vi "Screen_Vitreous.vi"(5 "File to Process":path) -> ()   [LabVIEW 2022 SP3]
uses:
  ViewData/-ReadEye/ScaleMethod.ctl
  <vilib>/Utility/miscctls.llb/LVOffsetAndMultiplierTypeDef.ctl
  <vilib>/Utility/miscctls.llb/LVRectTypeDef.ctl
  <vilib>/Utility/miscctls.llb/LVBoundsTypeDef.ctl
  <vilib>/Analysis/5stat.llb/RMS (DBL).vi
  <vilib>/Analysis/NI_AALPro.lvlib
panel:
  out "Current File#":i32
  out "Total #Files":i32
  in  "Next File in Dir?":bool caption="F1"
  in  "Prev File":bool caption="F2"
  in  "Delete File":bool caption="<Delete>"
  in  "Tab Control":enum32{"Images", "Misc"}(tab)
  out "dB":dbl[][](graph)
  out "Sector":dbl[][](graph)
  in  "Slide":cluster{dbl, dbl}(slide)={0.0, -48.10126582278481} scale=-80.0..-1.0
  in  "Comment Field (Optional)":string
  in  "Save Comment ?":bool
  in  "Type of Mean":u16(ring)=4 items=["Mean from lines", "Mean just lines", "Poly Mean", "No mean", "Filter"]
  in  "Filter Prams":T1={"low cutoff"=5, "order"=81, "high cutoff"=35}
  in  "Sound Speed":i16=1485
  out "RMS noise":dbl format="%#.2g"
  out "DynRange":dbl format="%#.2f"
  out "RF Window Pts":i32
  out "RF Lines":i32
  in  "Axis scaling":bool=TRUE
  in  "View Header?":bool
  in  "Alter Header":bool
  in  "Eye to BMP":bool
  in  "Display mode":T2=enum."dB Scale"
  out "Raw data":dbl[][](graph)
  out "Scan Info":T3
  in  "Create Sector":bool
  out "Axis scaling Params":T4 {"Y high" format="%.2f"; "Y low" format="%.2f"; "X left" format="%.2f"; "X right" format="%.2f"}
  out "cursor":dbl
  in  "Smooth factor":i32=1
  in  "Pixels in x":i16=170
  in  "Pixels in y":i16=1000
  in  "Reduce x data factor":i32=2
  out "inc x (mm)":dbl format="%.3f"
  out "inc y (mm)":dbl format="%.3f"
  in  "Add Lines":u16=1
  in  "File Ext":string="*.eye"
  in  "Save eye":bool
  in  "ExitSendCmd":bool
  # "For screening *.eye file stacks. Mainly meant for Aviso data acquired with custom digitizer set up."
  # "Push folder symbol to select first 'eye' to view in a folder.\nPress \"F1\" on keybard to increment up one image\nPress \"F2\" on keyboard to decrement down one image\nPress \"<Delete>\" on keyboard to delete a \"bad\" image\nSelect \"Save Comment\" to save any text that is entered into \"Comment Field\"\nExit program by pressing \"Stop\""
  # "© 2022 Weill Cornell Medicine"
  # "Crop sides with yellow line"
  # "Save sector as *.eye file in virtual RF space. Use add lines 4.\nPixels in y adjusts virtual sampling rate."
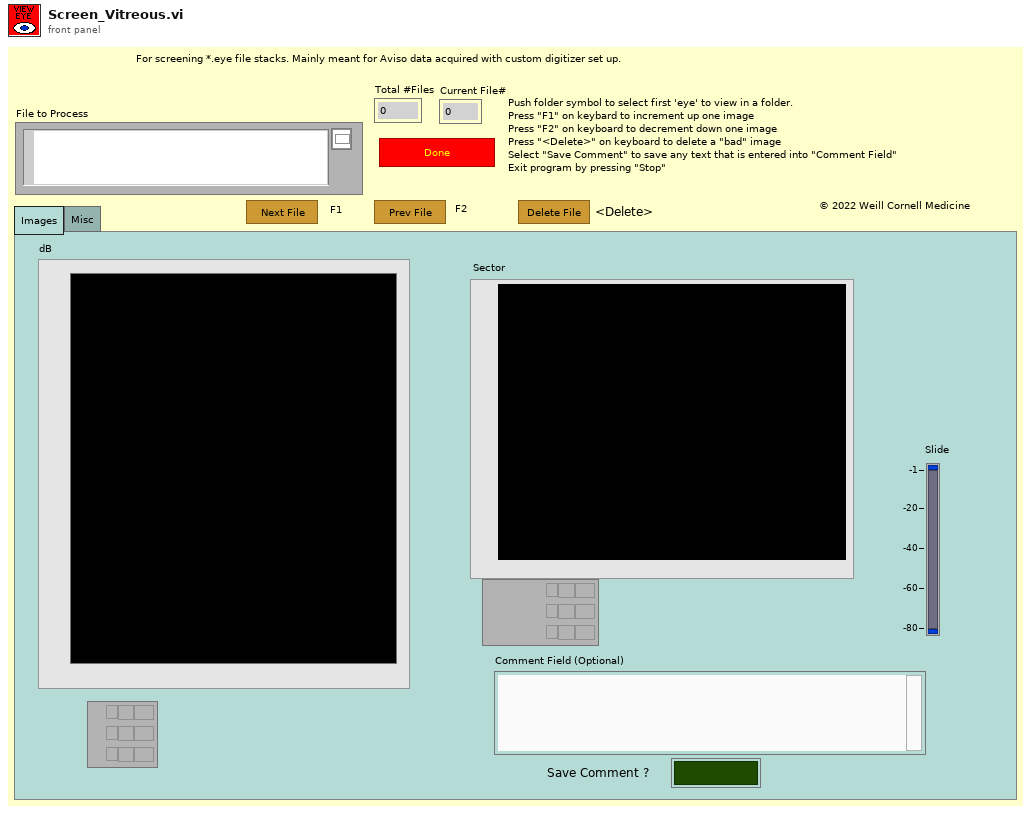
[diagram p1: front panel]
types:
  T1 = cluster{"low cutoff":i32, "order":i32, "high cutoff":i32}
  T2 = typedef "ScaleMethod.ctl" = enum16{"Linear Abs Grey", "Log Grey Scale", "Linear Color Scale", "dB Scale", "Verasonics Doppler"}
  T3 = cluster{"delay":sgl, "pivot distance":sgl, "sector scan angle":sgl, "operator":string, "Scan Mode":string, "location":string}
  T4 = cluster{"X right":dbl, "X left":dbl, "Y low":dbl, "Y high":dbl}
  T5 = enum16{"big-endian, network order", "native, host order", "little-endian"}
  T6 = enum16{"open", "replace", "create", "open or create", "replace or create", "replace or create with confirmation"}
  T7 = typedef "Header.ctl" = cluster{"header info":cluster{"Header":string, "Head length":i16}, "A/D info":cluster{"# rf points per line":u16, "# lines per scan":u16, "sample rate MHz":u16, "# A/D bits":i16, "# bytes per A/D":u16, "TGC Flag":u16, "A/D Type":string}, "Tranducer Info":cluster{"bandwidth":sgl, "center freq":sgl, "start freq":sgl, "ID":i32}, "Scan Info":cluster{"delay":sgl, "pivot distance":sgl, "sector scan angle":sgl, "operator":string, "Scan Mode":string, "location":string}, "Time/Date Info":cluster{"date":string, "time":string}, "RF Info":cluster{"RF file name":string, "RF file att":string, "RF cal file name":string, "RF cal file att":string}, "Patient Info":cluster{"ID":string, "extended ID":string, "age":u16, "sex":string, "previously\nscanned":string, "PSA":sgl, "LOS":u8, "Ethnicty 2":u8, "Race":u8}, "Tissue Type":cluster{"organ":i16, "disease type":i16, "disease location":i16, "IQ_pts":u16, "RcvBuffer":u8, "RcvFrame":u16, "IQBuff":u8, "IQFrame":u16, "IQPage":u8}, "Votage scaling":cluster{"Digitizer (dB)":sgl, "Gain (dB)":sgl, "Atten (dB)":sgl}, "Comment":string, "Misc Info":cluster{"avg num":u16, "c speed":i16, "Div By or SF zones":i16, "XMIT CHS":u8, "RCV CHS":u8, "Xmit angle":sgl}, "Therapy Parameters":cluster{"Theraputic Freq (MHz)":sgl, "Time on (s)":sgl, "Therapy amplitude (mV)":sgl, "Lines Before":u16, "Lines After":u16}, "Scan Settings":cluster{"Energy (uJ or V)":u8, "Damp (Ohm) or Fc":u8, "HP Filt (KHz)":u8, "LP Filt (MHz)":u8, "Gain (db)":u8, "prf (kHz)":sgl, "Distance between\nscan lines (um)":u16, "Distance between\nscan planes (um)":u16, "Scan line gap (um)":sgl, "Scan plane gap (um)":sgl}, "Compression Parameters":cluster{"F1 (MHz)":sgl, "F2 (MHz)":sgl, "% taper":sgl, "duration":sgl}, "Patient Info Xtra":cluster{"First Name":string, "Last Name":string, "Notes":string}, "ROI Box":u16[]}
  T8 = typedef "LVOffsetAndMultiplierTypeDef.ctl" = cluster{"Offset":dbl, "Multiplier":dbl}
  T9 = typedef "LVBoundsTypeDef.ctl" = cluster{"Width":u32, "Height":u32}
  T10 = typedef "LVRectTypeDef.ctl" = cluster{"Left":i16, "Top":i16, "Right":i16, "Bottom":i16}
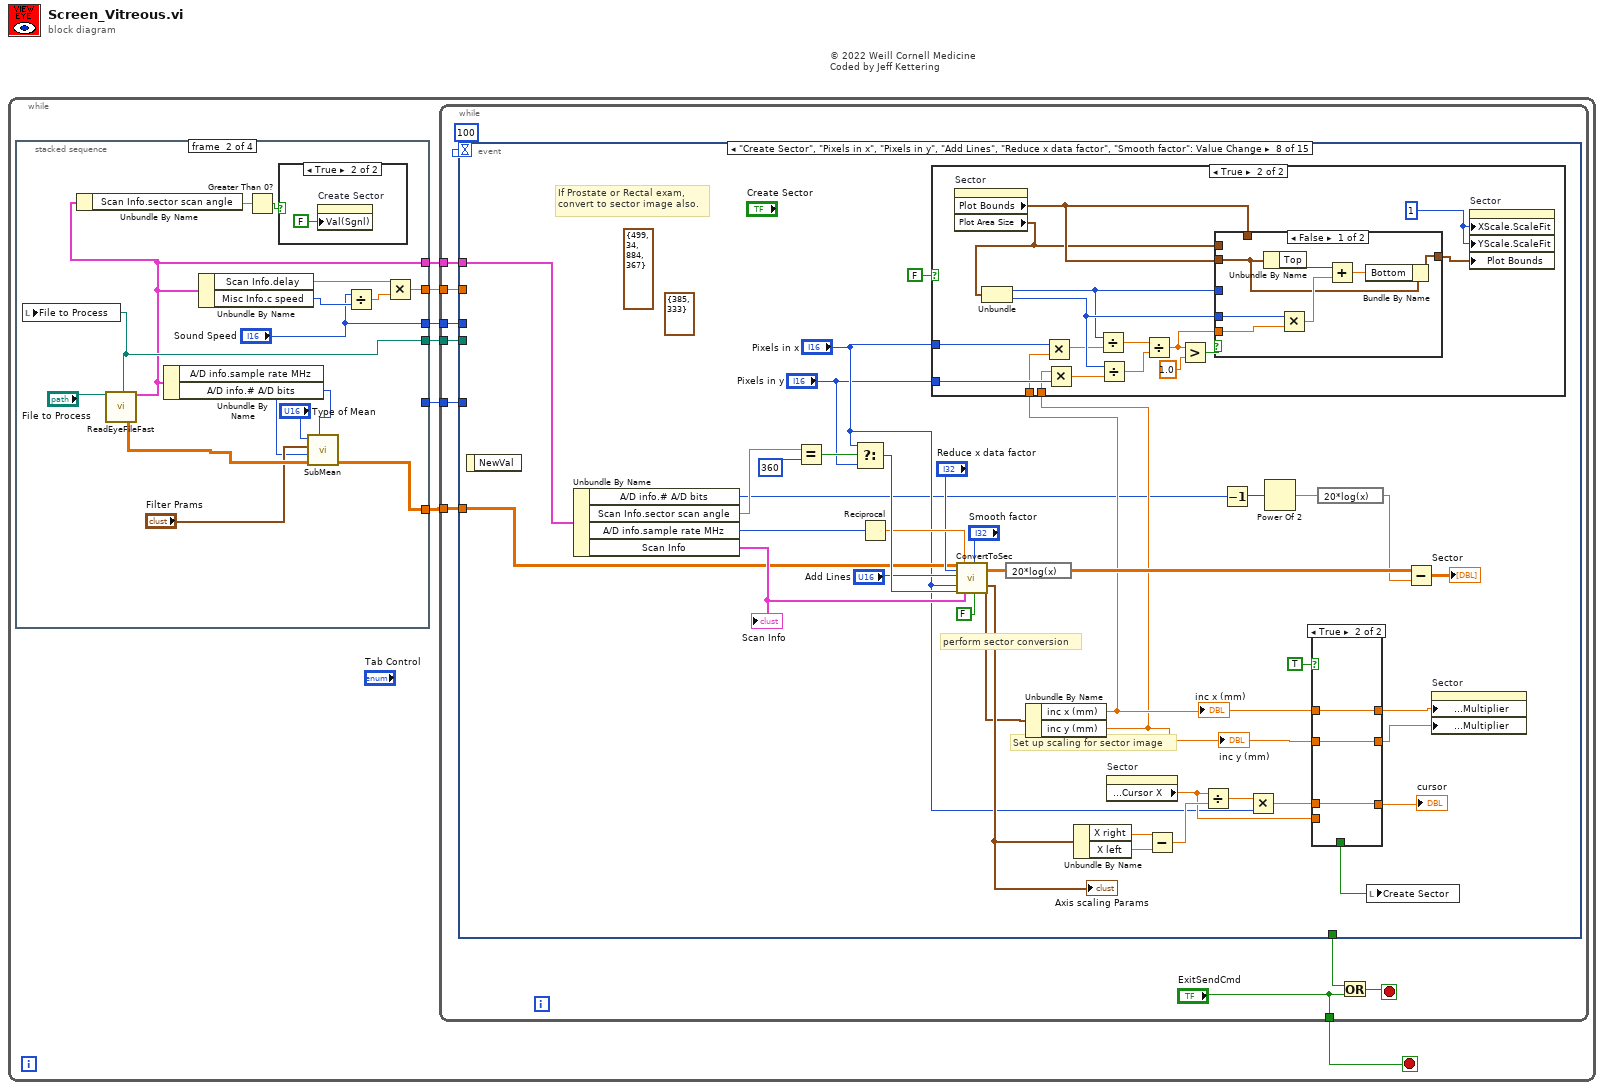
[diagram p0: block diagram]
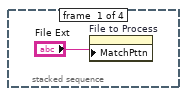
[diagram p2: hidden frame]
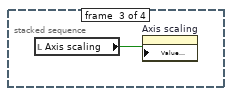
[diagram p4: hidden frame]
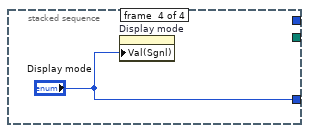
[diagram p5: hidden frame]
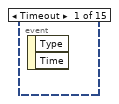
[diagram p6: hidden frame]
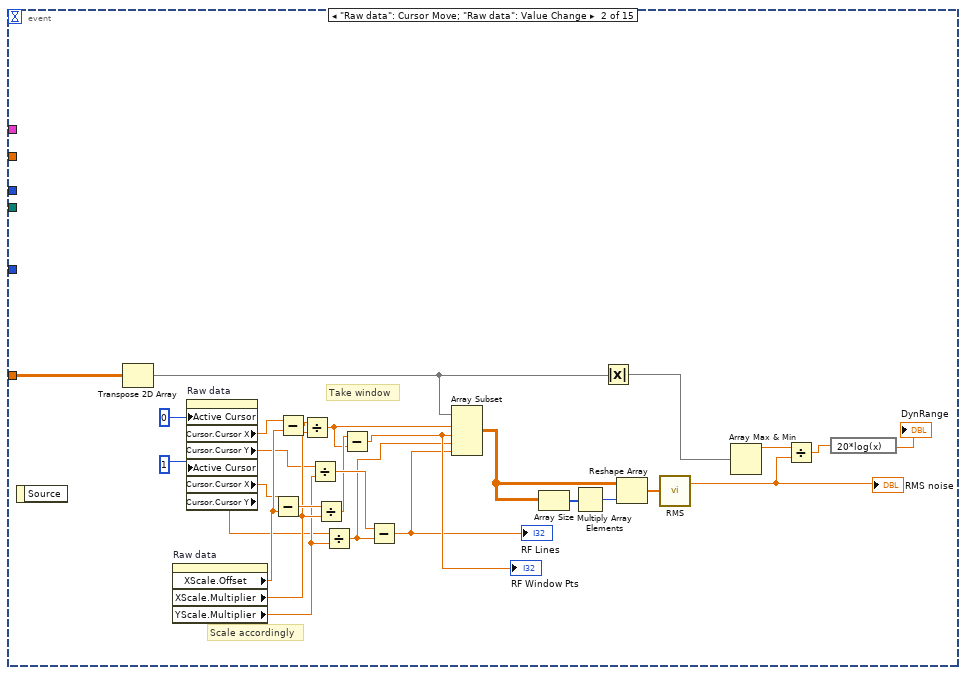
[diagram p7: hidden frame]
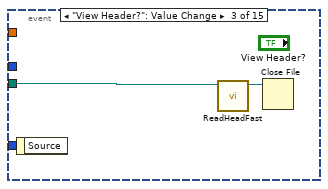
[diagram p8: hidden frame]
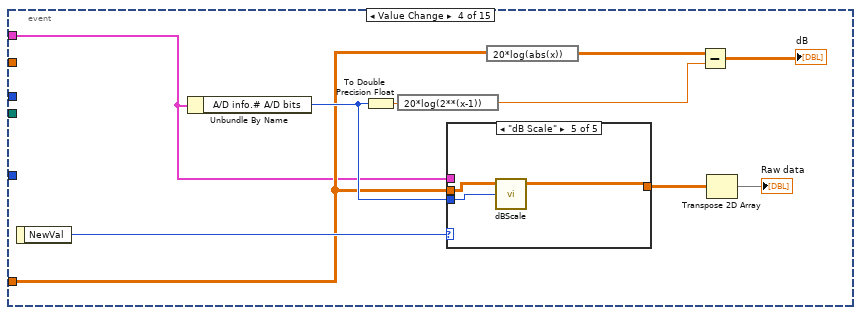
[diagram p9: hidden frame]
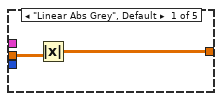
[diagram p10: hidden frame]
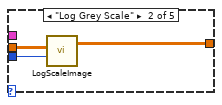
[diagram p11: hidden frame]
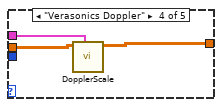
[diagram p13: hidden frame]
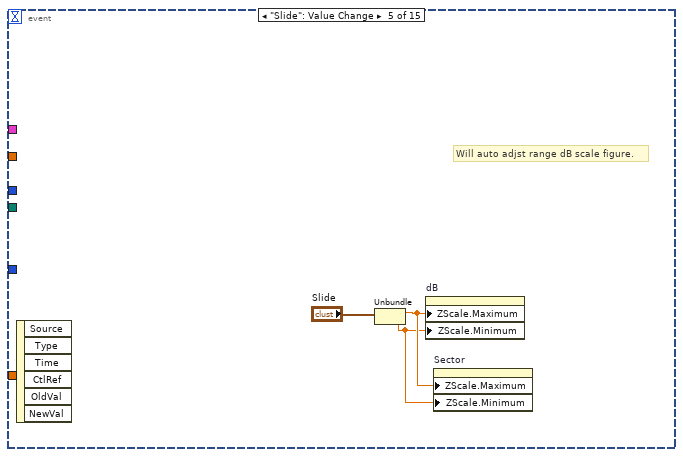
[diagram p14: hidden frame]
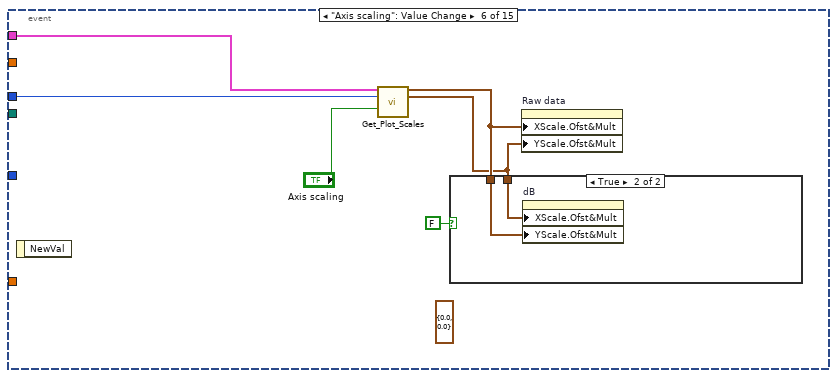
[diagram p15: hidden frame]
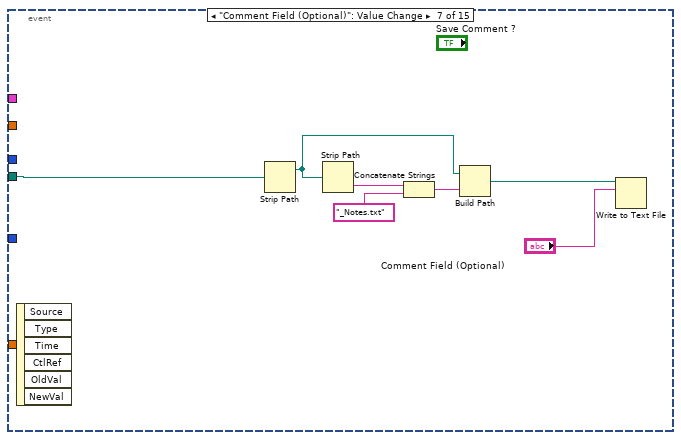
[diagram p17: hidden frame]
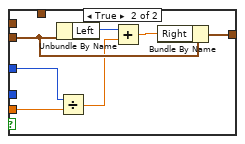
[diagram p19: hidden frame]
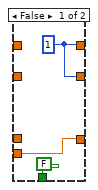
[diagram p20: hidden frame]
diagram:
  # "© 2022 Weill Cornell Medicine\nCoded by Jeff Kettering"
  n1 = while {
    stop <- w6 stop-if-true
    n2 = stacked-sequence {
      tunnel: [_ w22 _ _] -> w7
      tunnel: [_ w24 _ _] -> w5
      tunnel: [_ _ _ "Display mode"] -> w4
      tunnel: [_ w10 _ _] -> w3
      tunnel: [_ w15 _ _] -> w2
      tunnel: [_ "Sound Speed" _ _] -> w1
      frame #0 {
        n3 = property on="File to Process" class="Path"("MatchPttn"="File Ext") -> ()  [unwired: 2 in, 2 out]
      }
      frame #1 {
        n4 = call "ReadEyeFileFast.vi"("new file path"="File to Process") -> ("new path out"=w24:path, "2-D data array"=w23:sgl[][], "Header In"=w10:T7)  [unwired: 1 in, 15 out]
        n5 = local write "File to Process"(w24) -> ()
        n6 = Unbundle By Name(w10) -> ("Scan Info.sector scan angle"=w11:sgl)
        n7 = Unbundle By Name(w10) -> ("A/D info.sample rate MHz"=w13:u16, "A/D info.# A/D bits"=w9:i16)
        n8 = Unbundle By Name(w10) -> ("Scan Info.delay"=w16:sgl, "Misc Info.c speed"=w18:i16)
        n9 = Greater Than 0?(x=w11) -> (x > 0?=w12:bool)
        n10 = case shown="True" w12 {
          frame False {
          }
          frame True {
            n11 = property on="Create Sector" class="Bool (strict)"("Val(Sgnl)"=FALSE ("Value (Signaling)")) -> ()  [unwired: 2 in, 2 out]
          }
        }
        n12 = call "SubMean.vi"("Bit Depth"=w9, "Scan Data In"=w23, "Samp Rate (MHz)"=w13, "Filter Prams"="Filter Prams", "Type of Mean"="Type of Mean") -> ("Array"=w22:dbl[][])  [unwired: 1 in, 2 out]
        n13 = Divide(x="Sound Speed", y=w18) -> (x/y=w17:dbl)
        n14 = Multiply(x=w16, y=w17) -> (x*y=w15:dbl)
      }
      frame #2 {
        n15 = local read "Axis scaling"() -> (w26:bool)
        n16 = property on="Axis scaling" class="Bool (strict)"("Value (Signaling)"=w26) -> ()  [unwired: 2 in, 2 out]
      }
      frame #3 {
        n17 = property on="Display mode" class="Enum (strict)"("Val(Sgnl)"="Display mode") -> ()  [unwired: 2 in, 2 out]
      }
    }
    n18 = while {
      tunnel: w7 -> [w37]
      tunnel: w5 -> [w35]
      tunnel: w4 -> [w34]
      tunnel: ["ExitSendCmd"] -> w6
      tunnel: w3 -> [w30]
      tunnel: w2 -> [w29]
      tunnel: w1 -> [w28]
      stop <- w31 stop-if-true
      n19 = event shown="[7] \"Create Sector\", \"Pixels in x\", \"Pixels in y\", \"Add Lines\", \"Reduce x data factor\", \"Smooth factor\": Value Change" {
        selector: _ -> [_ _ _ _ _ _ _ _ _ _ _ _ _ _ _]
        dyn-events: _ -> [_ _ _ _ _ _ _ _ _ _ _ _ _ _ _]
        timeout: 100 -> [_ _ _ _ _ _ _ _ _ _ _ _ _ _ _]
        tunnel: w37 -> [_ w57 _ w72 _ _ _ w118 w226 _ _ _ _ _ _]
        tunnel: w35 -> [_ _ w67 _ _ _ w107 _ w205 _ w246 w294 w307 w309 _]
        tunnel: w34 -> [_ _ _ _ _ _ _ _ _ _ _ _ _ _ _]
        tunnel: [_ _ _ _ _ _ _ _ _ TRUE TRUE TRUE TRUE _ TRUE] -> w32
        tunnel: w30 -> [_ _ _ w70 _ w96 _ w131 w215 _ _ _ _ _ _]
        tunnel: w29 -> [_ _ _ _ _ _ _ _ _ _ _ _ _ _ _]
        tunnel: w28 -> [_ _ _ _ _ w97 _ _ _ _ _ _ _ _ _]
        event Timeout {
          n20 = event-data() -> ()  [unwired: 3 out]
        }
        event "Raw data": Cursor Move; "Raw data": Value Change {
          # "Take window"
          # "Scale accordingly"
          n21 = event-data() -> ()  [unwired: 2 out]
          n22 = Transpose 2D Array(2D array=w57) -> (transposed array=w42:dbl[][])
          n23 = property on="Raw data" class="IntGraph (strict)"() -> ("XScale.Offset"=w56:dbl, "XScale.Multiplier"=w55:dbl, "YScale.Multiplier"=w54:dbl)  [unwired: 2 in, 2 out]
          n24 = property on="Raw data" class="IntGraph (strict)"("Active Cursor"=u32 0 ("Write Attribute"), "Active Cursor"=u32 1 ("Write Attribute")) -> ("Cursor.Cursor X"=w53:dbl, "Cursor.Cursor Y"=w49:dbl, "Cursor.Cursor X"=w52:dbl, "Cursor.Cursor Y"=w48:dbl)  [unwired: 2 in, 2 out]
          n25 = Subtract(x=w52, y=w56) -> (x-y=w59:dbl)
          n26 = Subtract(x=w53, y=w56) -> (x-y=w60:dbl)
          n27 = Divide(x=w60, y=w55) -> (x/y=w47:dbl)
          n28 = Divide(x=w49, y=w54) -> (x/y=w61:dbl)
          n29 = Divide(x=w59, y=w55) -> (x/y=w58:dbl)
          n30 = Divide(x=w48, y=w54) -> (x/y=w45:dbl)
          n31 = Subtract(x=w58, y=w47) -> (x-y=w46:dbl)
          "RF Window Pts" <- w46
          n32 = Subtract(x=w61, y=w45) -> (x-y=w44:dbl)
          "RF Lines" <- w44
          n33 = Array Subset(array=w42, index (row)=w47, length (row)=w46, index (col)=w45, length (col)=w44) -> (w39:dbl[][])
          n34 = Array Size(array=w39) -> (size(s)=w64:i32[])
          n35 = Multiply Array Elements(1:w64) -> (0:w62:i32)
          n36 = Absolute Value(x=w42) -> (abs(x)=w43:dbl[][])
          n37 = Reshape Array(w39, w62) -> (w63:dbl[])
          n38 = call-poly <vilib>:"RMS.vi"("X"=w63) -> ("rms value"=w38:dbl)  [unwired: 1 out]
          "RMS noise" <- w38
          n39 = Array Max & Min(array=w43) -> (max value=w65:dbl)  [unwired: 3 out]
          n40 = Divide(x=w65, y=w38) -> (x/y=w40:dbl)
          n41 = expression code="20*log(x)"(w40) -> (→"DynRange":dbl)
        }
        event "View Header?": Value Change {
          n42 = event-data() -> ()  [unwired: 2 out]
          n43 = call "ReadHeadFast.vi"("new file path"=w67) -> ("refnum out"=w66:refnum<file>)  [unwired: 7 in, 3 out]
          n44 = Close File(refnum=w66) -> ()  [unwired: 1 in, 2 out]
        }
        event Value Change {
          n45 = event-data() -> ("NewVal"=w76:T2)  [unwired: 1 out]
          n46 = Unbundle By Name(w70) -> ("A/D info.# A/D bits"=w75:i16)
          n47 = To Double Precision Float(number=w75) -> (double precision float=w74:dbl)
          n48 = expression code="20*log(2**(x-1))"(w74) -> (w73:dbl)
          n49 = case shown="\"dB Scale\"" w76 {
            tunnel: [w78 w82 w83 w85 w88] -> w69
            tunnel: w72 -> [w79 w81 w83 w86 w89]
            tunnel: w75 -> [_ w80 _ _ w87]
            tunnel: w70 -> [_ _ _ w84 _]
            frame "Linear Abs Grey", Default {
              n50 = Absolute Value(x=w79) -> (abs(x)=w78:dbl[][])
            }
            frame "Log Grey Scale" {
              n51 = call "LogScaleImage.vi"("A/D bits"=w80, "input array"=w81) -> ("log scale image"=w82:dbl[][])  [unwired: 1 out]
            }
            frame "Linear Color Scale" {
            }
            frame "Verasonics Doppler" {
              n52 = call "DopplerScale.vi"("Header In"=w84, "Velocity index in"=w86) -> ("Velocity Out"=w85:dbl[][])  [unwired: 6 in, 3 out]
            }
            frame "dB Scale" {
              n53 = call "dBScale.vi"("Bit Depth"=w87, "Data In"=w89) -> ("Data Out"=w88:dbl[][])  [unwired: 3 in]
            }
          }
          n54 = expression code="20*log(abs(x))"(w72) -> (w71:dbl[][])
          n55 = Subtract(x=w71, y=w73) -> (x-y=→"dB":dbl[][])
          n56 = Transpose 2D Array(2D array=w69) -> (transposed array=→"Raw data":dbl[][])
        }
        event "Slide": Value Change {
          # "Will auto adjst range dB scale figure."
          n57 = event-data() -> ()  [unwired: 7 out]
          n58 = Unbundle("Slide") -> (w91:dbl, w90:dbl)
          n59 = property on="dB" class="IntGraph (strict)"("ZScale.Maximum"=w91, "ZScale.Minimum"=w90) -> ()  [unwired: 2 in, 2 out]
          n60 = property on="Sector" class="IntGraph (strict)"("ZScale.Maximum"=w91, "ZScale.Minimum"=w90) -> ()  [unwired: 2 in, 2 out]
        }
        event "Axis scaling": Value Change {
          (unwired) T8 {"Offset"=0.0, "Multiplier"=0.0} ("X Scale.Offset and Multiplier")
          n61 = event-data() -> ()  [unwired: 2 out]
          n62 = call "Get_Plot_Scales.vi"("Header In"=w96, "Sound Speed modify"=w97, "Axis scaling"="Axis scaling") -> ("Depth Scale"=w95:cluster{"start depth":dbl, "depth interval":dbl}, "Width Scale"=w94:cluster{"Start":dbl, "width Interval":dbl})  [unwired: 11 in]
          n63 = case shown="True" FALSE {
            tunnel: w95 -> [_ w100]
            tunnel: w94 -> [_ w99]
            frame False {
            }
            frame True {
              n64 = property on="dB" class="IntGraph (strict)"("XScale.Ofst&Mult"=w99, "YScale.Ofst&Mult"=w100) -> ()  [unwired: 2 in, 2 out]
            }
          }
          n65 = property on="Raw data" class="IntGraph (strict)"("XScale.Ofst&Mult"=w95, "YScale.Ofst&Mult"=w94) -> ()  [unwired: 2 in, 2 out]
        }
        event "Comment Field (Optional)": Value Change {
          n66 = event-data() -> ()  [unwired: 7 out]
          n67 = Strip Path(path=w107) -> (stripped path=w101:path)  [unwired: 1 out]
          n68 = Strip Path(path=w101) -> (name=w106:string)  [unwired: 1 out]
          n69 = Concatenate Strings(w106, "_Notes.txt" ("search string")) -> (w102:string)
          n70 = Build Path(base path=w101, name or relative path=w102) -> (appended path=w104:path)
          n71 = Write to Text File(file (use dialog)=w104, text="Comment Field (Optional)") -> ()  [unwired: 2 in, 3 out]
        }
        event "Create Sector", "Pixels in x", "Pixels in y", "Add Lines", "Reduce x data factor", "Smooth factor": Value Change {
          (unwired) T9 {"Width"=385, "Height"=333} ("Plot Area:Size")
          (unwired) T10 {"Left"=499, "Top"=34, "Right"=884, "Bottom"=367} ("Plot Area Bounds")
          # "Set up scaling for sector image"
          # "If Prostate or Rectal exam,\nconvert to sector image also."
          # "perform sector conversion"
          n72 = event-data() -> ()  [unwired: 2 out]
          n73 = Unbundle By Name(w131) -> ("A/D info.# A/D bits"=w110:i16, "Scan Info.sector scan angle"=w123:sgl, "A/D info.sample rate MHz"=w124:u16, "Scan Info"=w130:T3)
          "Scan Info" <- w130
          n74 = Equal?(x=w123, y=360) -> (x = y?=w143:bool)
          n75 = Select(t="Pixels in x", s=w143, f="Pixels in y") -> (s? t:f=w145:i16)
          n76 = Reciprocal(x=w124) -> (1/x=w142:dbl)
          n77 = call "ConvertToSec.vi"("raw image data in"=w118, "reduce pts by factor of"="Reduce x data factor", "Add Lines"="Add Lines", "pixels in x"="Pixels in x", "pixels in y"=w145, "Time between rf pts\nmicros"=w142, "Scan Info"=w130, "Smooth factor"="Smooth factor", "use min z value?"=FALSE) -> ("raw sector out"=w121:dbl[][], "Axis scaling Params"=w132:T4, "scales"=w128:cluster{"inc x (mm)":dbl, "inc y (mm)":dbl})  [unwired: 3 in, 5 out]
          "Axis scaling Params" <- w132
          n78 = expression code="20*log(x)"(w121) -> (w120:dbl[][])
          n79 = Unbundle By Name(w128) -> ("inc x (mm)"=w115:dbl, "inc y (mm)"=w114:dbl)
          "inc y (mm)" <- w114
          "inc x (mm)" <- w115
          n80 = case shown="True" FALSE {
            tunnel: "Pixels in x" -> [_ w153]
            tunnel: "Pixels in y" -> [_ w152]
            tunnel: w115 -> [_ w151]
            tunnel: w114 -> [_ w150]
            frame False {
            }
            frame True {
              w148 = u8 1 ("X Scale.Scale Fit")
              n81 = property on="Sector" class="IntGraph (strict)"() -> ("Plot Bounds"=w147:T10, "Plot Area Size"=w146:T9)  [unwired: 2 in, 2 out]
              n82 = Unbundle(w146) -> ("Width"=w160:u32, "Height"=w162:u32)
              n83 = Multiply(x=w153, y=w151) -> (x*y=w154:dbl)
              n84 = Multiply(x=w150, y=w152) -> (x*y=w155:dbl)
              n85 = Divide(x=w160, y=w154) -> (x/y=w156:dbl)
              n86 = Divide(x=w162, y=w155) -> (x/y=w157:dbl)
              n87 = Divide(x=w156, y=w157) -> (x/y=w161:dbl)
              n88 = Greater?(x=w161, y=1.0) -> (0:w158:bool)
              n89 = case shown="False" w158 {
                tunnel: w160 -> [_ w176]
                tunnel: w161 -> [w169 w175]
                tunnel: w162 -> [w168 _]
                tunnel: w147 -> [w163 w174]
                tunnel: [w164 w170] -> w149
                tunnel: w147 -> [_ _]
                tunnel: w146 -> [_ _]
                frame False {
                  n90 = Unbundle By Name(w163) -> ("Top"=w167:i16)
                  n91 = Multiply(x=w168, y=w169) -> (x*y=w165:dbl)
                  n92 = Add(x=w167, y=w165) -> (x+y=w166:dbl)
                  n93 = Bundle By Name(cluster=w163, "Bottom"=w166) -> (w164:T10)
                }
                frame True {
                  n94 = Unbundle By Name(w174) -> ("Left"=w172:i16)
                  n95 = Divide(x=w176, y=w175) -> (x/y=w173:dbl)
                  n96 = Add(x=w172, y=w173) -> (x+y=w171:dbl)
                  n97 = Bundle By Name(cluster=w174, "Right"=w171) -> (w170:T10)
                }
              }
              n98 = property on="Sector" class="IntGraph (strict)"("XScale.ScaleFit"=w148, "YScale.ScaleFit"=w148, "Plot Bounds"=w149) -> ()  [unwired: 2 in, 2 out]
            }
          }
          n99 = Unbundle By Name(w132) -> ("X right"=w141:dbl, "X left"=w140:dbl)
          n100 = property on="Sector" class="IntGraph (strict)"() -> ("Cursor.Cursor Position:Cursor X"=w134:dbl)  [unwired: 2 in, 2 out]
          n101 = Subtract(x=w141, y=w140) -> (x-y=w139:dbl)
          n102 = Divide(x=w134, y=w139) -> (x/y=w138:dbl)
          n103 = Decrement(x=w110) -> (x-1=w112:i16)
          n104 = Multiply(x=w138, y="Pixels in x") -> (x*y=w135:dbl)
          n105 = Power Of 2(x=w112) -> (2^x=w111:dbl)
          n106 = case shown="True" TRUE {
            tunnel: w115 -> [_ w182]
            tunnel: [w179 w182] -> w137
            tunnel: [w179 w181] -> w136
            tunnel: w114 -> [_ w181]
            tunnel: w135 -> [_ w180]
            tunnel: [w178 w180] -> w133
            tunnel: w134 -> [w178 _]
            tunnel: [FALSE ("Create Sector") _] -> w119
            frame False {
              w179 = 1
            }
            frame True {
            }
          }
          "cursor" <- w133
          n107 = expression code="20*log(x)"(w111) -> (w109:dbl)
          n108 = local write "Create Sector"(w119) -> ()
          n109 = Subtract(x=w120, y=w109) -> (x-y=→"Sector":dbl[][])
          n110 = property on="Sector" class="IntGraph (strict)"("X Scale.Offset and Multiplier:Multiplier"=w137, "Y Scale.Offset and Multiplier:Multiplier"=w136) -> ()  [unwired: 2 in, 2 out]
        }
        event "Save eye": Value Change {
          w207 = FALSE ("prepend array or string size? (T)")
          w214 = sgl 0.0 ("Scan Info.pivot distance")
          # "Set up scaling for sector image"
          # "perform sector conversion"
          n111 = event-data() -> ()  [unwired: 7 out]
          n112 = Unbundle By Name(w215) -> ("Scan Info.sector scan angle"=w227:sgl, "A/D info.sample rate MHz"=w228:u16, "Scan Info"=w231:T3, "Misc Info.c speed"=w197:i16)
          n113 = local read "Pixels in y"() -> (w225:i16)
          n114 = local read "Pixels in x"() -> (w211:i16)
          n115 = Equal?(x=w227, y=360) -> (x = y?=w234:bool)
          n116 = Select(t=w211, s=w234, f=w225) -> (s? t:f=w210:i16)
          n117 = Reciprocal(x=w228) -> (1/x=w233:dbl)
          n118 = Strip Path(path=w205) -> (stripped path=w190:path, name=w204:string)
          n119 = local read "Add Lines"() -> (w223:u16)
          n120 = local read "Reduce x data factor"() -> (w224:i32)
          n121 = local read "Smooth factor"() -> (w191:i32)
          n122 = call "ConvertToSec.vi"("raw image data in"=w226, "reduce pts by factor of"=w224, "Add Lines"=w223, "pixels in x"=w211, "pixels in y"=w210, "Time between rf pts\nmicros"=w233, "Scan Info"=w231, "Abs?"=FALSE, "Interp Mode"=2, "Smooth factor"=w191, "use min z value?"=FALSE) -> ("raw sector out"=w206:dbl[][], "Axis scaling Params"=w232:T4, "scales"=w229:cluster{"inc x (mm)":dbl, "inc y (mm)":dbl})  [unwired: 1 in, 5 out]
          n123 = Search and Replace String(input string=w204, search string=".eye" ("input string"), replace string="Sec.eye" ("replace string (\"\")")) -> (result string=w203:string)  [unwired: 5 in, 3 out]
          n124 = Build Path(base path=w190, name or relative path="Sector" ("replace string (\"\")")) -> (appended path=w187:path)
          n125 = Unbundle By Name(w229) -> ("inc x (mm)"=w199:dbl, "inc y (mm)"=w196:dbl)
          n126 = Unbundle By Name(w232) -> ("Y high"=w213:dbl)
          n127 = Absolute Value(x=w213) -> (abs(x)=w212:dbl)
          n128 = Divide(x=w197, y=w196) -> (x/y=w195:dbl)
          n129 = expression code="x*1000"(w199) -> (w198:dbl)
          n130 = call <vilib>:"Check if File or Folder Exists.vi"("path"=w187) -> ("file or folder exists?"=w188:bool, "dup path"=w185:path)  [unwired: 8 in, 1 out]
          n131 = expression code="x/2000"(w195) -> (w194:dbl)
          n132 = case shown="False" w188 {
            tunnel: [w237 w238] -> w186
            tunnel: w185 -> [w236 w238]
            frame False {
              n133 = Create Folder(path (use dialog)=w236) -> (created path=w237:path)  [unwired: 2 in, 2 out]
            }
            frame True {
            }
          }
          n134 = Bundle By Name(cluster=w215, "A/D info.# rf points per line"=w210, "A/D info.# lines per scan"=w211, "Scan Info.delay"=w212, "Scan Info.pivot distance"=w214, "Scan Info.sector scan angle"=w214, "Scan Settings.Distance between\nscan lines (um)"=w198, "A/D info.sample rate MHz"=w194) -> (w209:T7)
          n135 = To Word Integer(number=w206) -> (16bit integer=w193:i16[][])
          n136 = Build Path(base path=w186, name or relative path=w203) -> (appended path=w200:path)
          n137 = Open/Create/Replace File(file path (use dialog)=w200, operation (0:open)=T6."replace or create") -> (refnum out=w220:refnum<file>, error out=w219:errorcluster)  [unwired: 4 in, 1 out]
          n138 = call "MakeHeader.vi"("Header In"=w209) -> ("Header String"=w208:string)  [unwired: 6 in]
          n139 = Write to Binary File(file (use dialog)=w220, data=w208, error in=w219, 5:w207) -> (refnum out=w222:refnum<file>, error out=w221:errorcluster)  [unwired: 2 in, 1 out]
          n140 = Write to Binary File(file (use dialog)=w222, data=w193, error in=w221, 5:w207, 9:T5."little-endian" ("byte order (0:big-endian, network order)")) -> (refnum out=w217:refnum<file>, error out=w216:errorcluster)  [unwired: 1 in, 1 out]
          n141 = Close File(refnum=w217, error in=w216) -> ()  [unwired: 2 out]
        }
        event "File to Process", "File Ext": Value Change {
          n142 = event-data() -> ()  [unwired: 7 out]
        }
        event "Next File in Dir?", "Delete File": Value Change {
          # "Increment by one file in directory"
          n143 = event-data() -> ()  [unwired: 7 out]
          n144 = property on="File to Process" class="Path"() -> ("MatchPttn"=w248:string)  [unwired: 2 in, 2 out]
          n145 = Strip Path(path=w246) -> (stripped path=w242:path, name=w255:string)
          n146 = local write "Next File in Dir?"(FALSE ("Next File in Dir?")) -> ()
          n147 = List Folder(path=w242, pattern=w248) -> (path out=w247:path, filenames=w241:string[])  [unwired: 1 in, 3 out]
          n148 = Search 1D Array(1D array=w241, element=w255) -> (index of element=w254:i32)  [unwired: 1 out]
          n149 = Increment(x=w254) -> (x+1=w253:i32)
          "Current File#" <- w253
          n150 = Index Array(array=w241, index=w253) -> (element=w252:string)
          n151 = Array Size(array=w241) -> (size(s)=→"Total #Files":i32)
          n152 = Build Path(base path=w247, name or relative path=w252) -> (appended path=w244:path)
          n153 = case shown="True" "Delete File" {
            tunnel: w246 -> [_ w261]
            tunnel: w244 -> [_ _]
            frame False {
            }
            frame True {
              n154 = Strip Path(path=w261) -> (stripped path=w268:path, name=w264:string)
              n155 = Strip Path(path=w268) -> (stripped path=w267:path, name=w265:string)
              n156 = Build Path(base path=w267, name or relative path="Deleted Files" ("replace string (\"\")")) -> (appended path=w258:path)
              n157 = Strip Path(path=w261) -> (stripped path=w271:path, name=w275:string)
              n158 = Create Folder(path (use dialog)=w258) -> (created path=w257:path)  [unwired: 2 in, 2 out]
              n159 = Search and Replace String(input string=w275, search string=".eye", replace string=".bmp" ("replace string (\"\")")) -> (result string=w272:string)  [unwired: 5 in, 3 out]
              n160 = Build Path(base path=w257, name or relative path=w265) -> (appended path=w260:path)
              n161 = Create Folder(path (use dialog)=w260) -> (created path=w259:path)  [unwired: 2 in, 2 out]
              n162 = Build Path(base path=w271, name or relative path=w272) -> (appended path=w269:path)
              n163 = Build Path(base path=w259, name or relative path=w264) -> (appended path=w262:path)
              n164 = case shown="True" TRUE {
                tunnel: w261 -> [w276 w279]
                tunnel: w262 -> [_ w278]
                frame False {
                  n165 = Delete(path (use dialog)=w276, confirm (F)=FALSE) -> ()  [unwired: 1 in, 5 out]
                }
                frame True {
                  n166 = Move(source path=w279, 10:w278) -> ()  [unwired: 3 in, 3 out]
                }
              }
              n167 = Delete(path (use dialog)=w269, confirm (F)=FALSE) -> ()  [unwired: 1 in, 5 out]
            }
          }
          n168 = call <vilib>:"Check if File or Folder Exists.vi"("path"=w244) -> ("file or folder exists?"=w250:bool, "dup path"=w251:path)  [unwired: 1 in, 8 out]
          n169 = case shown="False" w250 {
            tunnel: w251 -> [_ w284]
            tunnel: w241 -> [w283 _]
            tunnel: w247 -> [w282 _]
            tunnel: [w280 w284] -> w249
            frame False {
              # "Handle last to first case"
              n170 = Index Array(array=w283) -> (element=w281:string)  [unwired: 1 in]
              n171 = Build Path(base path=w282, name or relative path=w281) -> (appended path=w280:path)
            }
            frame True {
            }
          }
          n172 = local write "File to Process"(w249) -> ()
        }
        event "Prev File": Value Change {
          n173 = event-data() -> ()  [unwired: 7 out]
          n174 = property on="File to Process" class="Path"() -> ("MatchPttn"=w286:string)  [unwired: 2 in, 2 out]
          n175 = Strip Path(path=w294) -> (stripped path=w298:path, name=w297:string)
          n176 = List Folder(path=w298, pattern=w286) -> (path out=w289:path, filenames=w288:string[])  [unwired: 1 in, 3 out]
          n177 = Search 1D Array(1D array=w288, element=w297) -> (index of element=w296:i32)  [unwired: 1 out]
          n178 = Decrement(x=w296) -> (x-1=w285:i32)
          n179 = Index Array(array=w288, index=w285) -> (element=w295:string)
          n180 = Build Path(base path=w289, name or relative path=w295) -> (appended path=w290:path)
          n181 = local write "Current File#"(w285) -> ()
          n182 = call <vilib>:"Check if File or Folder Exists.vi"("path"=w290) -> ("file or folder exists?"=w291:bool, "dup path"=w292:path)  [unwired: 1 in, 8 out]
          n183 = case shown="False" w291 {
            tunnel: w292 -> [_ w304]
            tunnel: w288 -> [w303 _]
            tunnel: w289 -> [w302 _]
            tunnel: [w300 w304] -> w287
            frame False {
              # "Handle first to last case"
              n184 = Reverse 1D Array(array=w303) -> (reversed array=w299:string[])
              n185 = Index Array(array=w299) -> (element=w301:string)  [unwired: 1 in]
              n186 = Build Path(base path=w302, name or relative path=w301) -> (appended path=w300:path)
            }
            frame True {
            }
          }
          n187 = local write "File to Process"(w287) -> ()
        }
        event "Alter Header": Value Change {
          n188 = event-data() -> ()  [unwired: 2 out]
          n189 = Strip Path(path=w307) -> (stripped path=w306:path)  [unwired: 1 out]
          n190 = call "AlterHeader.vi"("Choose Directory"=w306) -> ()  [unwired: 1 in, 2 out]
        }
        event "Eye to BMP": Value Change {
          n191 = event-data() -> ()  [unwired: 2 out]
          n192 = Strip Path(path=w309) -> (stripped path=w308:path)  [unwired: 1 out]
          n193 = call "MakeEyeBMP.vi"("Choose Directory"=w308) -> ()  [unwired: 15 out]
        }
        event "Type of Mean", "Filter Prams": Value Change {
          n194 = event-data() -> ()  [unwired: 7 out]
        }
      }
      n195 = Or(x=w32, y="ExitSendCmd") -> (x .or. y?=w31:bool)
    }
  }
